vi "PWM Output User Interface.vi"() -> ()   [LabVIEW 2023, in "GUI.lvlib" / "Diagnostic.lvlib"]
uses:
  Diagnostic.lvlib
  Control/PWM Output 6739.ctl
  Control/PWM Output.ctl
  Control/PWM Output 6612.ctl
  HardwareAbstractionLayer_LVOOP/PWM Output/NI PWM Output_class/NI PWM Output.lvclass
  D:/eDCU LTT/VT LTT Project/Source Code/HardwareAbstractionLayer_LVOOP/PWM Output/PWM Output_class/PWM Output.lvclass
  HardwareAbstractionLayer_LVOOP/Database/SQL Public VI/Control/DB Options.ctl
  HardwareAbstractionLayer_LVOOP/Main/Class Ref.ctl
  HardwareAbstractionLayer_LVOOP/DMM/DMM.lvclass
  HardwareAbstractionLayer_LVOOP/Function Generator/Function Generator.lvclass
  HardwareAbstractionLayer_LVOOP/Oscilloscope/Oscilloscope.lvclass
  HardwareAbstractionLayer_LVOOP/PowerSupply/PowerSupply.lvclass
  HardwareAbstractionLayer_LVOOP/Teststand/Teststand.lvclass
  HardwareAbstractionLayer_LVOOP/Analog Output/AO/AO.lvclass
  HardwareAbstractionLayer_LVOOP/Analog Input/AI/AI.lvclass
  HardwareAbstractionLayer_LVOOP/Database/Database.lvclass
  HardwareAbstractionLayer_LVOOP/Digital Output/DO_class/DO.lvclass
  HardwareAbstractionLayer_LVOOP/Digital Input/DI_class/DI.lvclass
  HardwareAbstractionLayer_LVOOP/PWM Output/PWM Output_class/PWM Output.lvclass
  HardwareAbstractionLayer_LVOOP/PWM Input/PWM Input_class/PWM Input.lvclass
  HardwareAbstractionLayer_LVOOP/NI Switch/NISwitch_class/NISwitch.lvclass
  HardwareAbstractionLayer_LVOOP/Modbus/Modbus_class/Modbus.lvclass
  HardwareAbstractionLayer_LVOOP/CAN/CAN Lib/CAN_class/CAN.lvclass
  HardwareAbstractionLayer_LVOOP/Main/Main.lvclass
panel:
  in  "Stop Acquire":bool
  in  "Start Acquire":bool
  out "error out":errorcluster
  in  "error in":errorcluster
  in  "Operation":T1(tab)
  in  "PXIe - 6739 M1":T2
  in  "PXIe - 6739 M2":T2
  in  "PXIe - 6612 M1":T4
  in  "PXIe - 6612 M2":T4
  in  "Stop":bool caption="Blank"
  # "PWM Output"
  # "Device:"
  # "***Note:  Duty Cycle Max Values Is 0.99 Only"
  # "Frequency"
  # "Dutycycles"
  # "Terminal Configuration"
  # "Enabled"
  # "Physical Channel"
  # "Frequency"
  # "Dutycycles"
  # "Terminal Configuration"
  # "Enabled"
  # "Physical Channel"
  # "Frequency"
  # "Dutycycles"
  # "Terminal Configuration"
  # "Enabled"
  # "Physical Channel"
  # "Frequency"
  # "Dutycycles"
  # "Terminal Configuration"
  # "Enabled"
  # "Physical Channel"
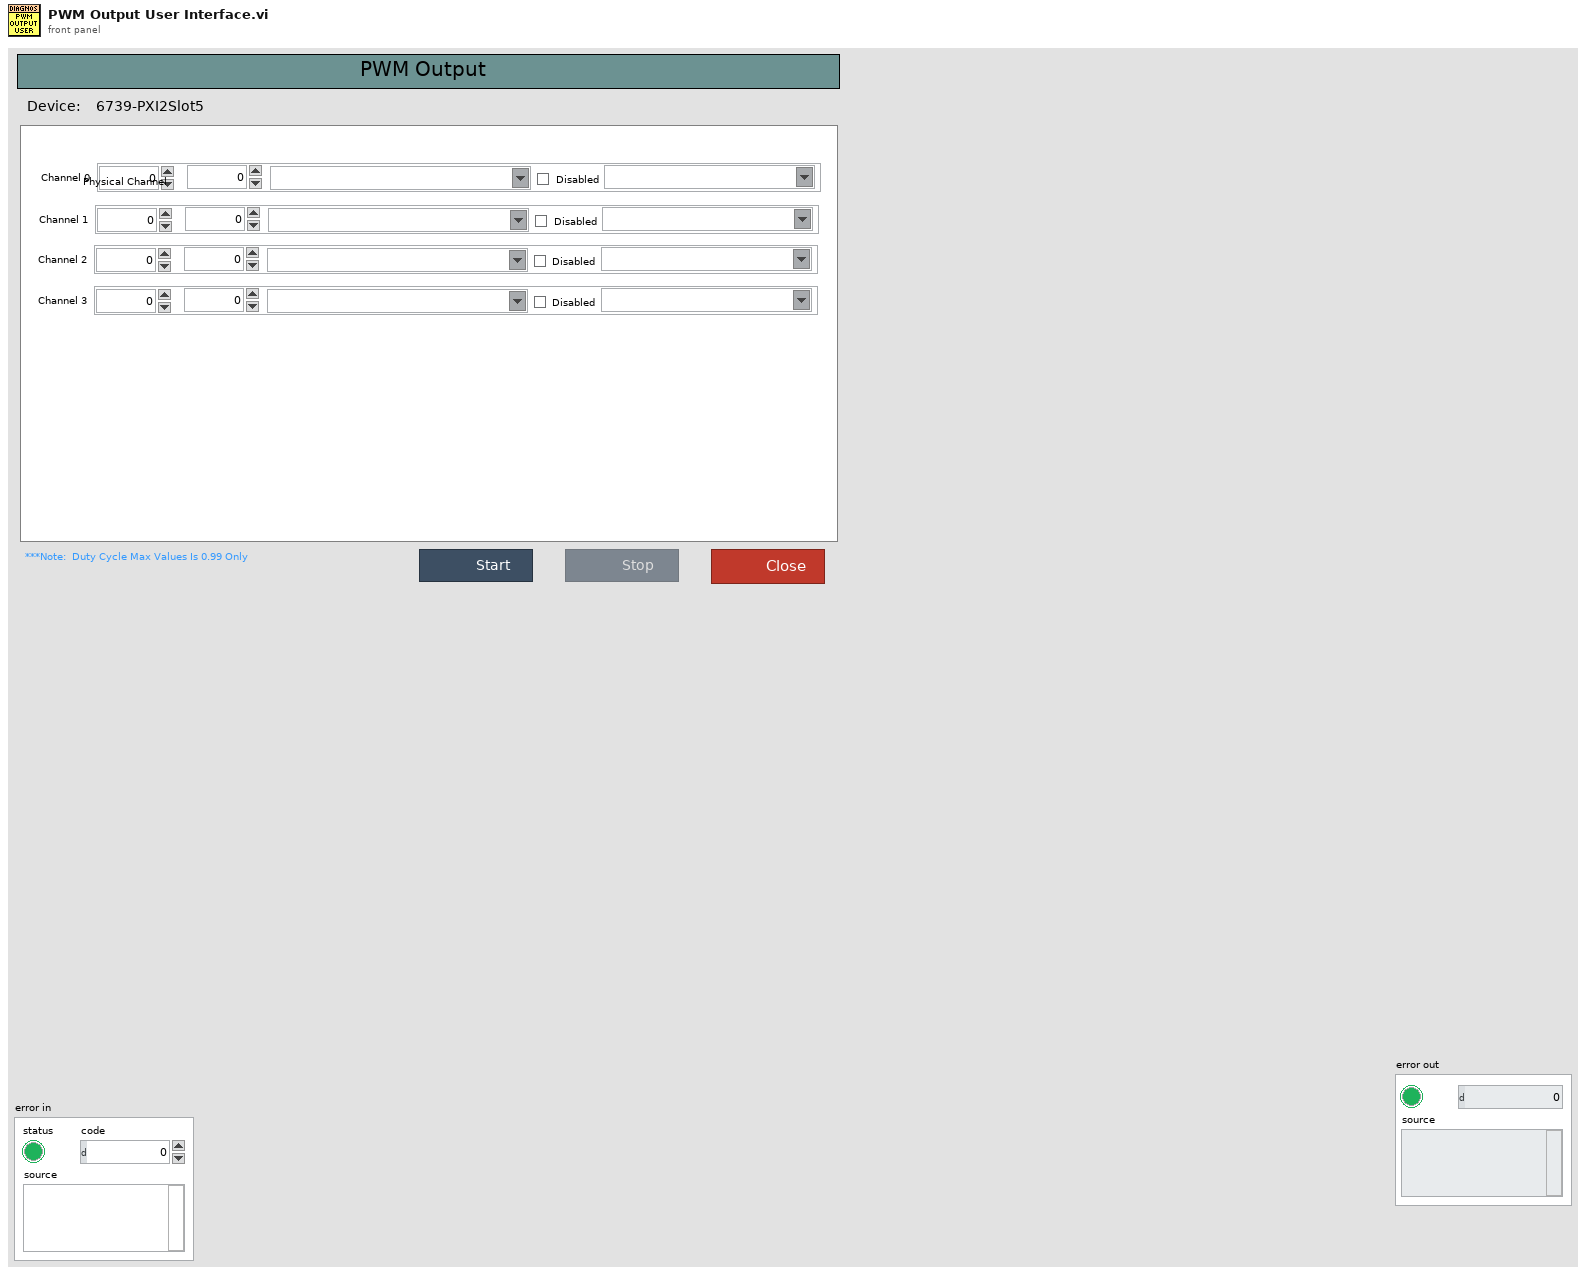
[diagram p1: front panel]
types:
  T1 = enum32{"6739-PXI2Slot5", "6739-PXI2Slot6", "6612-PXI2Slot7", "6612-PXI2Slot8"}
  T2 = typedef "GUI.lvlib/Diagnostic.lvlib/PWM Output 6739.ctl" = cluster{"Channel 0":T3, "Channel 1":T3, "Channel 2":T3, "Channel 3":T3}
  T3 = typedef "GUI.lvlib/Diagnostic.lvlib/PWM Output.ctl" = cluster{"Frequency":dbl, "Duty Cycles":dbl, "Terminal":tag, "Enable":bool, "Physical Channel":tag}
  T4 = typedef "GUI.lvlib/Diagnostic.lvlib/PWM Output 6612.ctl" = cluster{"Channel 0":T3, "Channel 1":T3, "Channel 2":T3, "Channel 3":T3, "Channel 4":T3, "Channel 5":T3, "Channel 6":T3, "Channel 7":T3}
  T5 = typedef "HardwareAbstractionLayer_LVOOP.lvlib/Database.lvclass/DB Options.ctl" = enum16{"Init", "Select Data", "Insert Data", "Update Data", "Delete Data", "Execute Query", "Create Schema", "Create Table", "List Tables", "List Columns", "Close"}
  T6 = typedef "HardwareAbstractionLayer_LVOOP.lvlib/Main.lvclass/Class Ref.ctl" = cluster{"DMM":refnum<class "DMM.lvclass">, "Function Generator":refnum<class "Function Generator.lvclass">, "Oscilloscope":refnum<class "Oscilloscope.lvclass">, "PowerSupply":refnum<class "PowerSupply.lvclass">, "Teststand":refnum<class "Teststand.lvclass">, "AO":refnum<class "AO.lvclass">, "AI":refnum<class "AI.lvclass">, "Database":refnum<class "Database.lvclass">, "AO Waveform Generation":refnum<class "AO.lvclass">, "DO":refnum<class "DO.lvclass">, "DI":refnum<class "DI.lvclass">, "PWM Output":refnum<class "PWM Output.lvclass">, "PWM Input":refnum<class "PWM Input.lvclass">, "RelayOutput":refnum<class "NISwitch.lvclass">, "Modbus":refnum<class "Modbus.lvclass">, "CAN":refnum<class "CAN.lvclass">}
  T7 = enum8{"Enabled", "Disabled", "Disabled and Grayed Out"}
  T8 = cluster{"[0]":T3, "[1]":T3, "[2]":T3, "[3]":T3, "[4]":T3, "[5]":T3, "[6]":T3, "[7]":T3}
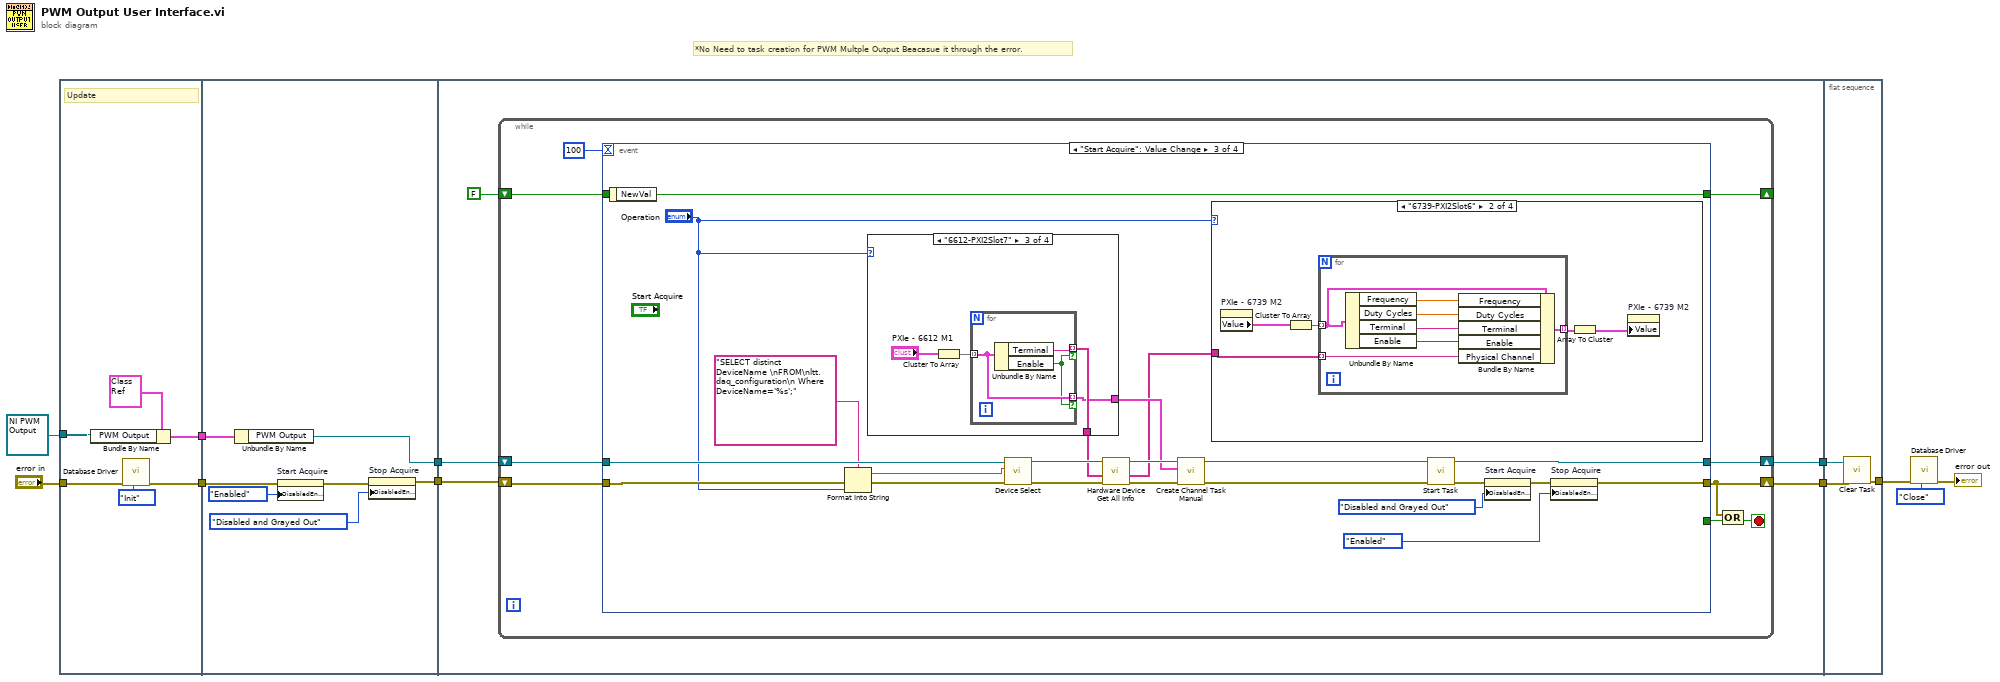
[diagram p0: block diagram]
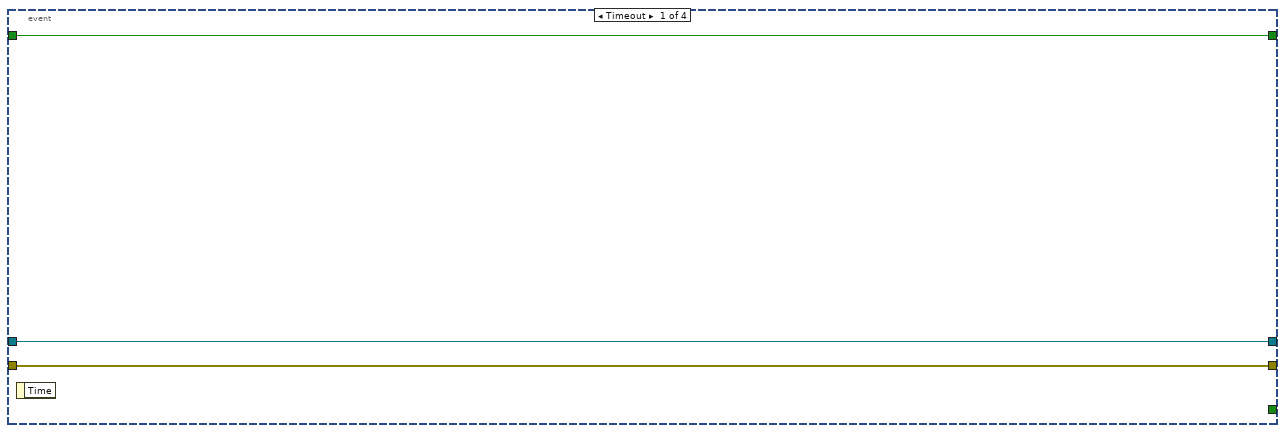
[diagram p2: hidden frame]
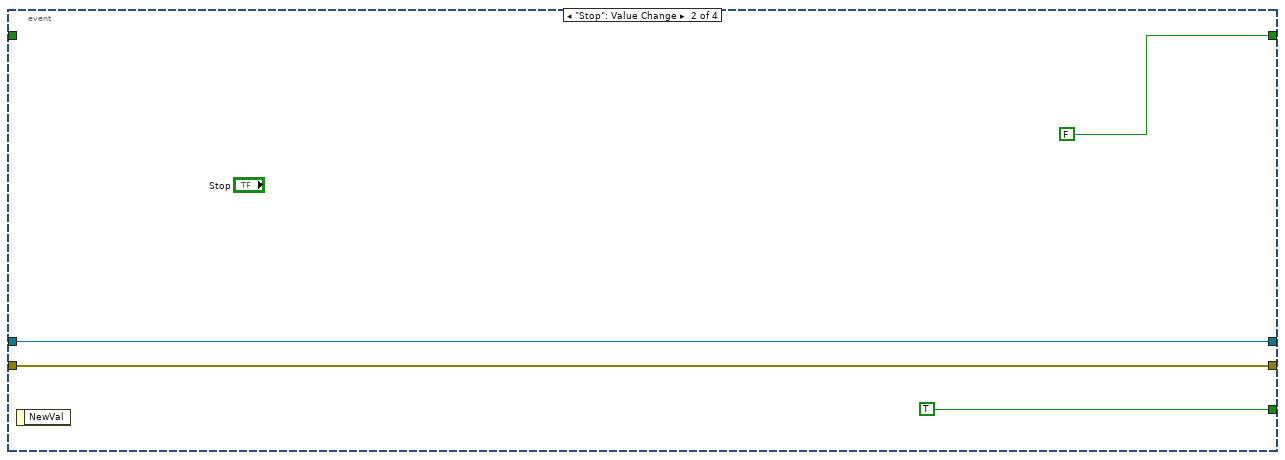
[diagram p3: hidden frame]
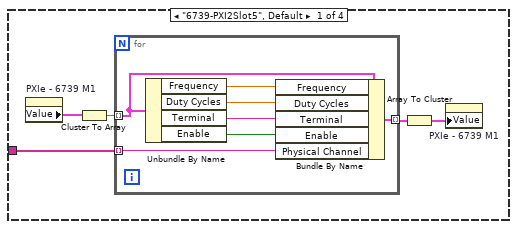
[diagram p4: hidden frame]
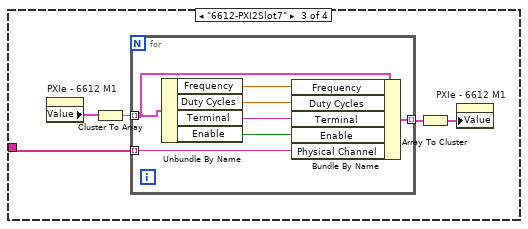
[diagram p5: hidden frame]
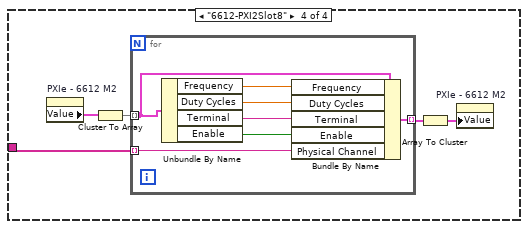
[diagram p6: hidden frame]
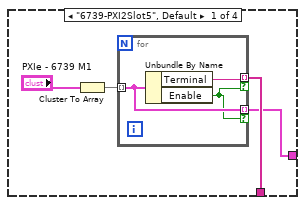
[diagram p7: hidden frame]
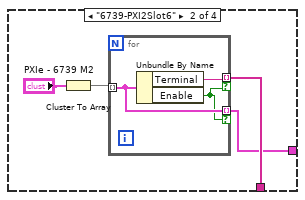
[diagram p8: hidden frame]
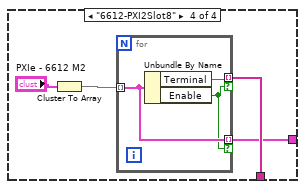
[diagram p9: hidden frame]
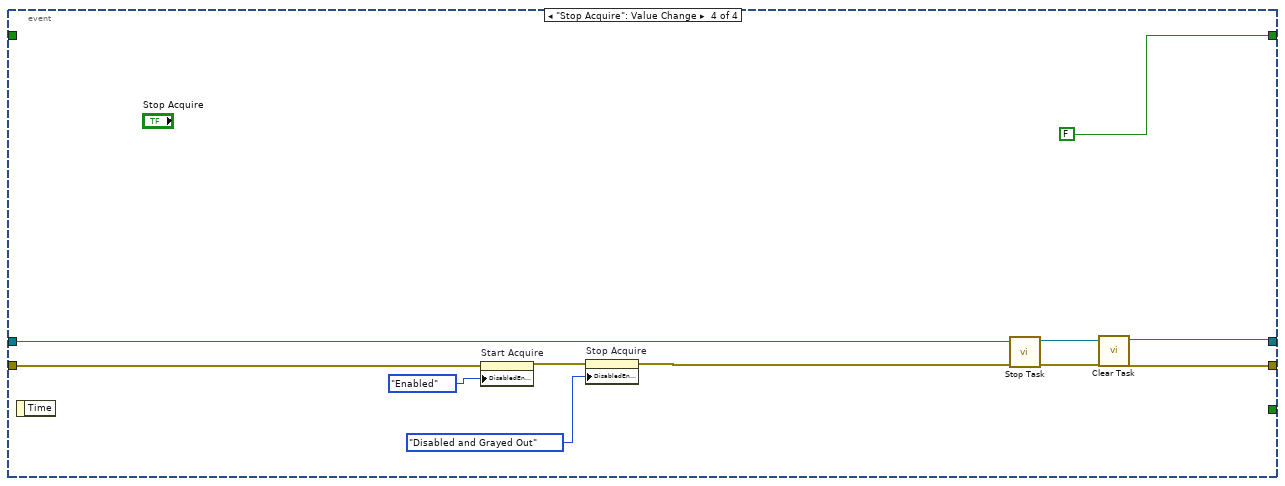
[diagram p10: hidden frame]
diagram:
  # "*No Need to task creation for PWM Multple Output Beacasue it through the error."
  n1 = flat-sequence {
    tunnel: "error in" -> [w17]
    tunnel: [w13] -> w10
    tunnel: [w15] -> w9
    tunnel: refnum<class "NI PWM Output.lvclass"> refnum ("HardwareAbstractionLayer_LVOOP.lvlib:NI PWM Output.lvclass") -> [w14]
    tunnel: w10 -> [w21]
    tunnel: w9 -> [w24]
    tunnel: [w23] -> w6
    tunnel: [w18] -> w1
    tunnel: w6 -> [w29]
    tunnel: [w28] -> w5
    tunnel: [w27] -> w4
    tunnel: w1 -> [w25]
    tunnel: [w155] -> w8
    tunnel: w5 -> [w157]
    tunnel: w4 -> [w156]
    frame #0 {
      # "Update"
      n2 = Bundle By Name(cluster=T6 {"DMM"=refnum, "Function Generator"=refnum, "Oscilloscope"=refnum, "PowerSupply"=refnum, "Teststand"=refnum, "AO"=refnum, "AI"=refnum, "Database"=refnum, "AO Waveform Generation"=refnum, "DO"=refnum, "DI"=refnum, "PWM Output"=refnum, "PWM Input"=refnum, "RelayOutput"=refnum, "Modbus"=refnum, "CAN"=refnum} ("Class Cluster"), "PWM Output"=w14) -> (w15:T6)
      n3 = call "Database Driver.vi"("Options"=DB_Options."Init", "error in"=w17) -> ("error out"=w13:errorcluster)  [unwired: 6 in, 3 out]
    }
    frame #1 {
      n4 = Unbundle By Name(w24) -> ("PWM Output"=w23:refnum<class "PWM Output.lvclass">)
      n5 = property on="Start Acquire" class="Bool"(error in=w21, "DisabledEnum"=T7."Enabled" ("Disabled")) -> (error out=w20:errorcluster)  [unwired: 1 in, 1 out]
      n6 = property on="Stop Acquire" class="Bool"(error in=w20, "DisabledEnum"=T7."Disabled and Grayed Out" ("Disabled")) -> (error out=w18:errorcluster)  [unwired: 1 in, 1 out]
    }
    frame #2 {
      n7 = while {
        shift-right: [w32] -> w27
        shift-left: w29 -> [w36]
        shift-right: [w33] -> w28
        shift-left: w25 -> [w35]
        shift-right: [w31] -> _
        shift-left: FALSE ("NewVal") -> [w30]
        stop <- w34 stop-if-true
        n8 = event shown="[2] \"Start Acquire\": Value Change" {
          selector: _ -> [_ _ _ _]
          dyn-events: _ -> [_ _ _ _]
          timeout: 100 -> [_ _ _ _]
          tunnel: [_ TRUE ("Stop") _ _] -> w37
          tunnel: [w40 w43 w54 w146] -> w33
          tunnel: w36 -> [w41 w44 w65 w150]
          tunnel: w35 -> [w40 w43 w49 w152]
          tunnel: [w41 w44 w56 w147] -> w32
          tunnel: [w39 FALSE ("NewVal") w58 FALSE ("NewVal")] -> w31
          tunnel: w30 -> [w39 _ _ _]
          event Timeout {
            n9 = event-data() -> ()  [unwired: 1 in, 1 out]
          }
          event "Stop": Value Change {
            n10 = event-data() -> ()  [unwired: 1 in, 1 out]
          }
          event "Start Acquire": Value Change {
            n11 = event-data() -> ("NewVal"=w58:bool)  [unwired: 1 in]
            n12 = Format Into String(format string="SELECT distinct DeviceName \nFROM\nltt.daq_configuration\n Where DeviceName='%s';" ("SQL query"), error in=w49, "Operation") -> (resulting string=w61:string, error out=w59:errorcluster)  [unwired: 1 in]
            n13 = case shown="\"6612-PXI2Slot7\"" "Operation" {
              tunnel: [w118 w124 w132 w139] -> w57
              tunnel: [w116 w123 w130 w137] -> w48
              frame "6739-PXI2Slot5", Default {
                n14 = Cluster To Array(cluster="PXIe - 6739 M1") -> (array=w117:T3[])
                n15 = for {
                  tunnel: w117 -> [w121] mode=indexing
                  tunnel: [w122] -> w118 mode=indexing if=w120
                  tunnel: [w121] -> w116 mode=indexing if=w120
                  n16 = Unbundle By Name(w121) -> ("Terminal"=w122:tag, "Enable"=w120:bool)
                }
              }
              frame "6739-PXI2Slot6" {
                n17 = Cluster To Array(cluster="PXIe - 6739 M2") -> (array=w125:T3[])
                n18 = for {
                  tunnel: w125 -> [w128] mode=indexing
                  tunnel: [w129] -> w124 mode=indexing if=w127
                  tunnel: [w128] -> w123 mode=indexing if=w127
                  n19 = Unbundle By Name(w128) -> ("Terminal"=w129:tag, "Enable"=w127:bool)
                }
              }
              frame "6612-PXI2Slot7" {
                n20 = Cluster To Array(cluster="PXIe - 6612 M1") -> (array=w131:T3[])
                n21 = for {
                  tunnel: [w136] -> w132 mode=indexing if=w134
                  tunnel: w131 -> [w135] mode=indexing
                  tunnel: [w135] -> w130 mode=indexing if=w134
                  n22 = Unbundle By Name(w135) -> ("Terminal"=w136:tag, "Enable"=w134:bool)
                }
              }
              frame "6612-PXI2Slot8" {
                n23 = Cluster To Array(cluster="PXIe - 6612 M2") -> (array=w138:T3[])
                n24 = for {
                  tunnel: [w143] -> w139 mode=indexing if=w141
                  tunnel: w138 -> [w142] mode=indexing
                  tunnel: [w142] -> w137 mode=indexing if=w141
                  n25 = Unbundle By Name(w142) -> ("Terminal"=w143:tag, "Enable"=w141:bool)
                }
              }
            }
            n26 = call-dynamic "Device Select.vi"("error in (no error)"=w59, "SQL query"=w61, "PWM Output in"=w65) -> ("error out"=w67:errorcluster, "PWM Output out"=w66:refnum<class "PWM Output.lvclass">)  [unwired: 7 in]
            n27 = call-dynamic "Hardware Device Get All Info.vi"("error in (no error)"=w67, "Terminals"=w57, "PWM Output in"=w66) -> ("error out"=w52:errorcluster, "CO.PhysicalChans"=w47:tag[], "PWM Output out"=w53:refnum<class "PWM Output.lvclass">)  [unwired: 6 in]
            n28 = call-dynamic "Create Channel Task Manual.vi"("error in (no error)"=w52, "Data"=w48, "PWM Output in"=w53) -> ("error out"=w51:errorcluster, "PWM Output out"=w50:refnum<class "PWM Output.lvclass">)  [unwired: 7 in]
            n29 = case shown="\"6739-PXI2Slot6\"" "Operation" {
              tunnel: w47 -> [w68 w82 w92 w104]
              frame "6739-PXI2Slot5", Default {
                n30 = property on="PXIe - 6739 M1" class="Clust (strict)"() -> ("Value"=w72:T2)  [unwired: 2 in, 2 out]
                n31 = Cluster To Array(cluster=w72) -> (array=w71:T3[])
                n32 = for {
                  tunnel: w71 -> [w79] mode=indexing
                  tunnel: [w75] -> w70 mode=indexing
                  tunnel: w68 -> [w73] mode=indexing
                  n33 = Unbundle By Name(w79) -> ("Frequency"=w78:dbl, "Duty Cycles"=w77:dbl, "Terminal"=w76:tag, "Enable"=w74:bool)
                  n34 = Bundle By Name(cluster=w79, "Frequency"=w78, "Duty Cycles"=w77, "Terminal"=w76, "Enable"=w74, "Physical Channel"=w73) -> (w75:T3)
                }
                n35 = Array To Cluster(array=w70) -> (cluster=w69:cluster{"[0]":T3, "[1]":T3, "[2]":T3, "[3]":T3})
                n36 = property on="PXIe - 6739 M1" class="Clust (strict)"("Value"=w69) -> ()  [unwired: 2 in, 2 out]
              }
              frame "6739-PXI2Slot6" {
                n37 = property on="PXIe - 6739 M2" class="Clust (strict)"() -> ("Value"=w81:T2)  [unwired: 2 in, 2 out]
                n38 = Cluster To Array(cluster=w81) -> (array=w84:T3[])
                n39 = for {
                  tunnel: w84 -> [w91] mode=indexing
                  tunnel: [w87] -> w83 mode=indexing
                  tunnel: w82 -> [w85] mode=indexing
                  n40 = Unbundle By Name(w91) -> ("Frequency"=w90:dbl, "Duty Cycles"=w89:dbl, "Terminal"=w88:tag, "Enable"=w86:bool)
                  n41 = Bundle By Name(cluster=w91, "Frequency"=w90, "Duty Cycles"=w89, "Terminal"=w88, "Enable"=w86, "Physical Channel"=w85) -> (w87:T3)
                }
                n42 = Array To Cluster(array=w83) -> (cluster=w80:cluster{"[0]":T3, "[1]":T3, "[2]":T3, "[3]":T3})
                n43 = property on="PXIe - 6739 M2" class="Clust (strict)"("Value"=w80) -> ()  [unwired: 2 in, 2 out]
              }
              frame "6612-PXI2Slot7" {
                n44 = property on="PXIe - 6612 M1" class="Clust (strict)"() -> ("Value"=w96:T4)  [unwired: 2 in, 2 out]
                n45 = Cluster To Array(cluster=w96) -> (array=w95:T3[])
                n46 = for {
                  tunnel: w95 -> [w103] mode=indexing
                  tunnel: [w99] -> w94 mode=indexing
                  tunnel: w92 -> [w97] mode=indexing
                  n47 = Unbundle By Name(w103) -> ("Frequency"=w102:dbl, "Duty Cycles"=w101:dbl, "Terminal"=w100:tag, "Enable"=w98:bool)
                  n48 = Bundle By Name(cluster=w103, "Frequency"=w102, "Duty Cycles"=w101, "Terminal"=w100, "Enable"=w98, "Physical Channel"=w97) -> (w99:T3)
                }
                n49 = Array To Cluster(array=w94) -> (cluster=w93:T8)
                n50 = property on="PXIe - 6612 M1" class="Clust (strict)"("Value"=w93) -> ()  [unwired: 2 in, 2 out]
              }
              frame "6612-PXI2Slot8" {
                n51 = property on="PXIe - 6612 M2" class="Clust (strict)"() -> ("Value"=w108:T4)  [unwired: 2 in, 2 out]
                n52 = Cluster To Array(cluster=w108) -> (array=w107:T3[])
                n53 = for {
                  tunnel: w107 -> [w115] mode=indexing
                  tunnel: [w111] -> w106 mode=indexing
                  tunnel: w104 -> [w109] mode=indexing
                  n54 = Unbundle By Name(w115) -> ("Frequency"=w114:dbl, "Duty Cycles"=w113:dbl, "Terminal"=w112:tag, "Enable"=w110:bool)
                  n55 = Bundle By Name(cluster=w115, "Frequency"=w114, "Duty Cycles"=w113, "Terminal"=w112, "Enable"=w110, "Physical Channel"=w109) -> (w111:T3)
                }
                n56 = Array To Cluster(array=w106) -> (cluster=w105:T8)
                n57 = property on="PXIe - 6612 M2" class="Clust (strict)"("Value"=w105) -> ()  [unwired: 2 in, 2 out]
              }
            }
            n58 = call-dynamic "Start Task.vi"("error in (no error)"=w51, "PWM Output in"=w50) -> ("error out"=w55:errorcluster, "PWM Output out"=w56:refnum<class "PWM Output.lvclass">)  [unwired: 8 in]
            n59 = property on="Start Acquire" class="Bool"(error in=w55, "DisabledEnum"=T7."Disabled and Grayed Out" ("Disabled")) -> (error out=w62:errorcluster)  [unwired: 1 in, 1 out]
            n60 = property on="Stop Acquire" class="Bool"(error in=w62, "DisabledEnum"=T7."Enabled" ("Disabled")) -> (error out=w54:errorcluster)  [unwired: 1 in, 1 out]
          }
          event "Stop Acquire": Value Change {
            n61 = event-data() -> ()  [unwired: 1 in, 1 out]
            n62 = property on="Start Acquire" class="Bool"(error in=w152, "DisabledEnum"=T7."Enabled" ("Disabled")) -> (error out=w151:errorcluster)  [unwired: 1 in, 1 out]
            n63 = property on="Stop Acquire" class="Bool"(error in=w151, "DisabledEnum"=T7."Disabled and Grayed Out" ("Disabled")) -> (error out=w144:errorcluster)  [unwired: 1 in, 1 out]
            n64 = call-dynamic "Stop Task.vi"("error in (no error)"=w144, "PWM Output in"=w150) -> ("error out"=w149:errorcluster, "PWM Output out"=w148:refnum<class "PWM Output.lvclass">)  [unwired: 8 in]
            n65 = call-dynamic "Clear Task.vi"("error in (no error)"=w149, "PWM Output in"=w148) -> ("error out"=w146:errorcluster, "PWM Output out"=w147:refnum<class "PWM Output.lvclass">)  [unwired: 8 in]
          }
        }
        n66 = Compound Arithmetic op=OR(w33, w37) -> (w34:bool)
      }
    }
    frame #3 {
      n67 = call-dynamic "Clear Task.vi"("error in (no error)"=w157, "PWM Output in"=w156) -> ("error out"=w155:errorcluster)  [unwired: 8 in, 1 out]
    }
  }
  n68 = call "Database Driver.vi"("Options"=DB_Options."Close", "error in"=w8) -> ("error out"=→"error out":errorcluster)  [unwired: 6 in, 3 out]
